vi "AOTF_Analog_Pulse_Switch.vi"(6 "Array 2":dbl[][](array[numeric]), 7 "Number of active lines":u8, 8 "AOTF-Analog out":T1, 9 "AOTF-Digital switch in":tag="/Dev1/PFI1", 10 "Pictures per pixel":u8, 11 "Pulse per Wavelength":u8[](array[numeric])) -> (0 "error out":errorcluster, 3 "task out":refnum<k21>)   [LabVIEW 2009]
uses:
  <vilib>/DAQmx/write.llb/DAQmx Write (Analog 2D DBL NChan NSamp).vi
  <vilib>/DAQmx/configure/timing.llb/DAQmx Timing (Sample Clock).vi
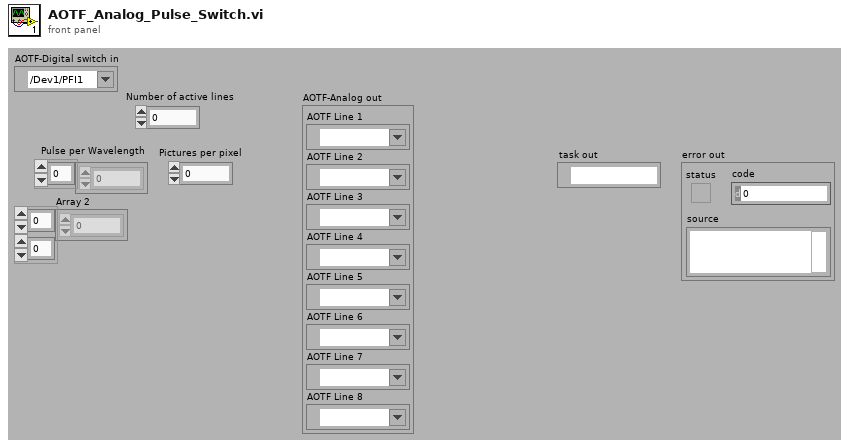
[diagram p1: front panel]
types:
  T1 = cluster{"AOTF Line 1":tag, "AOTF Line 2":tag, "AOTF Line 3":tag, "AOTF Line 4":tag, "AOTF Line 5":tag, "AOTF Line 6":tag, "AOTF Line 7":tag, "AOTF Line 8":tag}
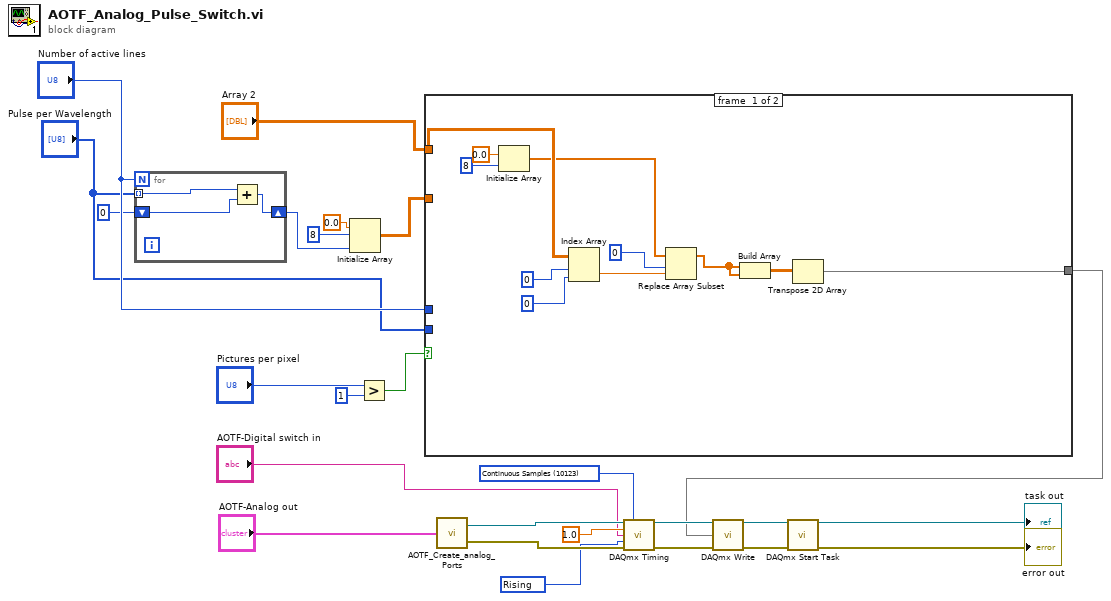
[diagram p0: block diagram]
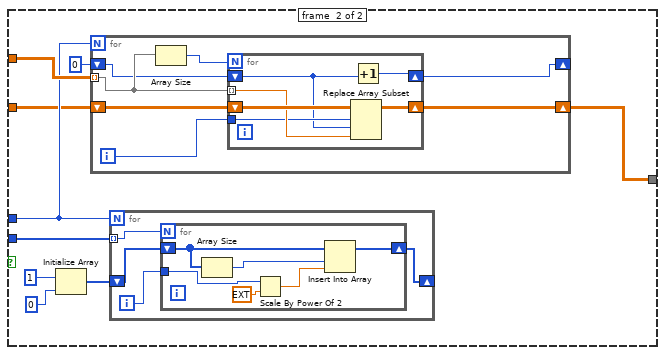
[diagram p2: hidden frame]
diagram:
  w22 = 10123 items=["Finite Samples"=10178, "Continuous Samples"=10123, "Hardware Timed Single Point"=12522] ("sample mode")
  w12 = 10280 items=["Rising"=10280, "Falling"=10171] ("active edge")
  n1 = for {
    N: "Number of active lines" -> [_]
    tunnel: "Pulse per Wavelength" -> [w26] mode=indexing
    shift-right: [w28] -> w3
    shift-left: 0 -> [w27]
    n2 = Add(x=w26, y=w27) -> (x+y=w28:i32)
  }
  n3 = Initialize Array(0.0 ("element"), 8 ("dimension size"), w3) -> (w6:dbl[][])
  n4 = Greater?(x="Pictures per pixel", y=u8 1) -> (0:w23:bool)
  n5 = case shown="True" w23 {
    tunnel: "Number of active lines" -> [_ w43]
    tunnel: "Pulse per Wavelength" -> [_ w48]
    tunnel: "Array 2" -> [w37 w44]
    tunnel: [w33 w41] -> w9
    tunnel: w6 -> [_ w42]
    frame #0 {
      n6 = Initialize Array(0.0 ("element"), 8 ("dimension size")) -> (w29:dbl[])
      n7 = Index Array(array=w37, index (row)=0, index (col)=0 ("disabled index (col)")) -> (element=w36:dbl)
      n8 = Replace Array Subset(array=w29, new element=w36, index=0) -> (w32:dbl[])
      n9 = Build Array(w32, w32) -> (w34:dbl[][])
      n10 = Transpose 2D Array(2D array=w34) -> (transposed array=w33:dbl[][])
    }
    frame #1 {
      n11 = Initialize Array(1 ("element"), 0 ("dimension size")) -> (w47:i32[])
      n12 = for {
        N: w43 -> [_]
        tunnel: w44 -> [w52] mode=indexing
        shift-right: [w54] -> w41
        shift-left: w42 -> [w55]
        shift-right: [w50] -> _
        shift-left: 0 -> [w49]
        i -> [w53]
        n13 = Array Size(array=w52) -> (size(s)=w51:i32)
        n14 = for {
          N: w51 -> [_]
          shift-right: [w60] -> w54
          shift-left: w55 -> [w61]
          tunnel: w52 -> [w59] mode=indexing
          tunnel: w53 -> [w58]
          shift-right: [w57] -> w50
          shift-left: w49 -> [w56]
          n15 = Replace Array Subset(array=w61, new element=w59, index (row)=w58, index (col)=w56) -> (w60:dbl[][])
          n16 = Increment(x=w56) -> (x+1=w57:i32)
        }
      }
      n17 = for {
        N: w43 -> [_]
        tunnel: w48 -> [w65] mode=indexing
        shift-right: [w63] -> _
        shift-left: w47 -> [w64]
        i -> [w62]
        n18 = for {
          N: w65 -> [_]
          shift-right: [w71] -> w63
          shift-left: w64 -> [w70]
          tunnel: w62 -> [w67]
          n19 = Array Size(array=w70) -> (size(s)=w69:i32)
          n20 = Scale By Power Of 2(n=w67, x=ext 1.0) -> (x*2^n=w68:ext)
          n21 = Insert Into Array(array=w70, index=w69, new element=w68) -> (w71:i32[])
        }
      }
    }
  }
  n22 = call "AOTF_Create_analog_Ports.vi"("Cluster"="AOTF-Analog out") -> ("task out"=w21:refnum<k21>, "error out"=w20:errorcluster)
  n23 = call-poly <vilib>:"DAQmx Timing.vi"("task/channels in"=w21, "sample mode"=w22, "rate"=1.0, "source"="AOTF-Digital switch in", "active edge"=w12, "error in"=w20) -> ("task out"=w19:refnum<k21>, "error out"=w18:errorcluster)  [unwired: 1 in, 7 out]
  n24 = call-poly <vilib>:"DAQmx Write.vi"("task/channels in"=w19, "data"=w9, "error in"=w18) -> ("task out"=w17:refnum<k21>, "error out"=w16:errorcluster)  [unwired: 1 in, 10 out]
  n25 = call <vilib>:"DAQmx Start Task.vi"("task/channels in"=w17, "error in"=w16) -> ("task out"=→"task out":refnum<k21>, "error out"=→"error out":errorcluster)  [unwired: 12 out]
